vi "ArmSetpointIndex.vi"(8 "ArmCurrent":dbl format="%#_13g", 9 "Joystick Input":dbl format="%#_13g", 10 "On Bert?":bool=TRUE, 11 "Arm State":T1) -> (2 "Lock Setpoint as Current Height":bool, 3 "Setpoint":dbl)   [LabVIEW 2014]
uses:
  Typedefs/Arm States.ctl
panel:
  in  "Ernie Arm LUT":dbl[](array[numeric])=[0.0, -27.0, -4.0, 0.497, 11.7, 26.3, 44.2, 56.3, 87.1, -10.0, -1.4, 76.0]
  out "Travel Direction Up":bool
  in  "Bert Arm LUT":dbl[](array[numeric])=[0.0, -26.0, -5.0, 0.497, 11.7, 26.3, 43.0, 56.1, 86.0, -13.0, -1.4, 72.0]
  # "Arm Manual"
  # "Arm Manual"
  # "Ground"
  # "Ground"
  # "Step"
  # "Step"
  # "1 Tote"
  # "1 Tote"
  # "2 Tote"
  # "2 Tote"
  # "3 Tote"
  # "3 Tote"
  # "4 Tote"
  # "4 Tote"
  # "5 Tote"
  # "5 Tote"
  # "6 Tote"
  # "6 Tote"
  # "Flip Can Arm"
  # "Flip Can Arm"
  # "Grab Can in Auto"
  # "Grab Can in Auto"
  # "4 bar nudge"
  # "4 Bar nudge"
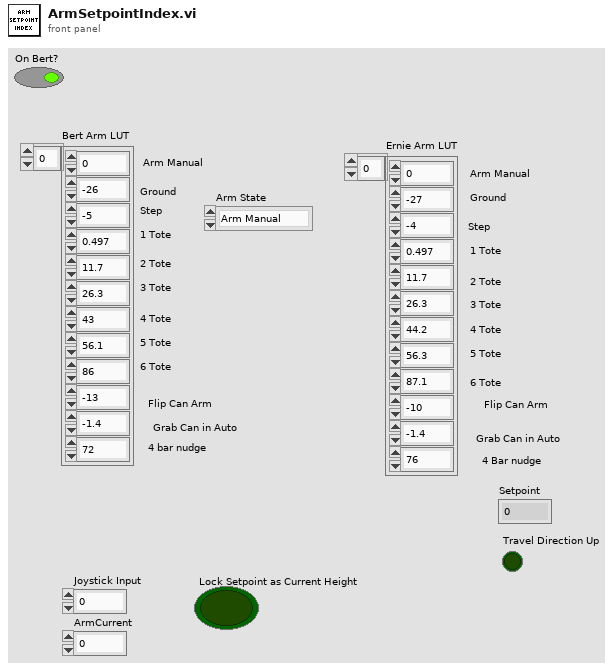
[diagram p1: front panel]
types:
  T1 = typedef "Arm States.ctl" = enum16{"Arm Manual ", "Ground", "Step", "1 Tote", "2 Tote", "3 Tote", "4 Tote", "5 Tote", "6 Tote", "Flip Can Arm", "Grab Can in auto", "Nudge"}
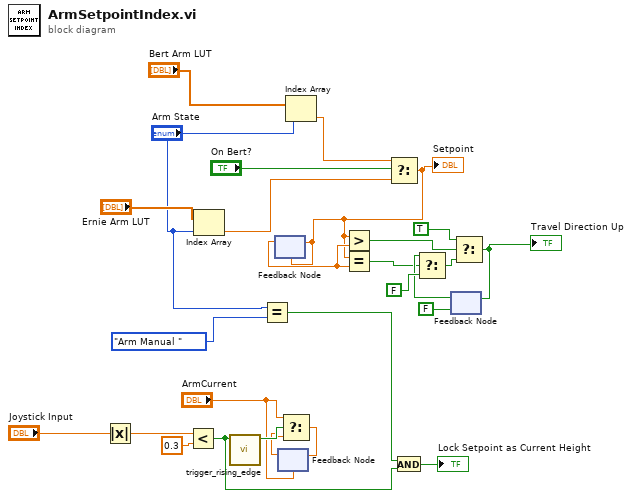
[diagram p0: block diagram]
diagram:
  n1 = Absolute Value(x="Joystick Input") -> (abs(x)=w10:dbl)
  n2 = Less?(x=w10, y=0.3) -> (x < y?=w4:bool)
  n3 = Index Array(array="Ernie Arm LUT", index="Arm State") -> (element=w15:dbl)
  n4 = call "trigger_rising_edge.vi"("input"=w4) -> ("rising"=w9:bool)  [unwired: 10 in]
  n5 = Equal?(x="Arm State", y=Arm_States."Arm Manual " ("Arm State")) -> (x = y?=w1:bool)
  n6 = feedback #1("ArmCurrent") -> (w8:dbl)
  n7 = Select(t="ArmCurrent", s=w9, f=w8) -> (s? t:f=w6:dbl)
  n8 = feedback-in #1(w6) -> ()
  n9 = Index Array(array="Bert Arm LUT", index="Arm State") -> (element=w16:dbl)
  n10 = Select(t=w16, s="On Bert?", f=w15) -> (s? t:f=w14:dbl)
  "Setpoint" <- w14
  n11 = feedback #2(w14) -> (w27:dbl)
  n12 = feedback-in #2(w14) -> ()
  n13 = Greater?(x=w14, y=w27) -> (0:w21:bool)
  n14 = Equal?(x=w14, y=w27) -> (x = y?=w24:bool)
  n15 = And(x=w1, y=w4) -> (x .and. y?=→"Lock Setpoint as Current Height":bool)
  n16 = feedback #3(FALSE) -> (w25:bool)
  n17 = Select(t=w25, s=w24, f=FALSE) -> (s? t:f=w23:bool)
  n18 = Select(t=TRUE, s=w21, f=w23) -> (s? t:f=w22:bool)
  "Travel Direction Up" <- w22
  n19 = feedback-in #3(w22) -> ()
